vi "TSM Get PSRR Settings.vi"(0 "TSM context":T1, 11 "error in (no error)":errorcluster) -> (3 "max V":dbl format="%#_13g", 4 "TSM context Out":T1, 6 "Sampling Rate (Hz)":dbl format="%#_13g", 8 "Samples per channel":i32=1000, 14 "min V":dbl format="%#_13g", 15 "error out":errorcluster)   [LabVIEW 2020]
doc: "Gets the PSRR settings from the specification file using TSM context"
uses:
  <vilib>/NI_TestStand_SemiconductorModule/NI_TestStand_Semiconductor_Module.lvlibp/PinMap/General/SemiconductorModuleContext.ctl
  <vilib>/NI_TestStand_SemiconductorModule/NI_TestStand_Semiconductor_Module.lvlibp/PinMap/Specs/NamespacedSymbolsToValues.vi
  <vilib>/NI_TestStand_SemiconductorModule/NI_TestStand_Semiconductor_Module.lvlibp
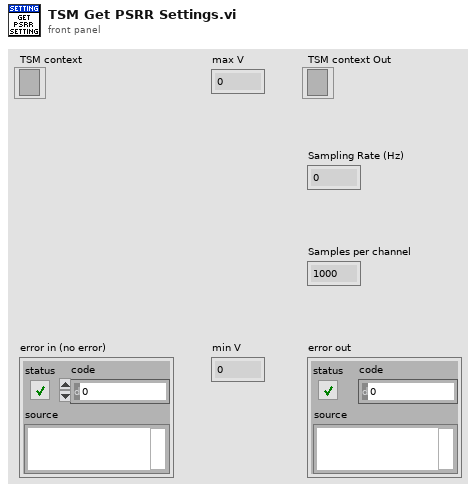
[diagram p1: front panel]
types:
  T1 = typedef "NI_TestStand_Semiconductor_Module.lvlibp/SemiconductorModuleContext.ctl" = refnum<k7>
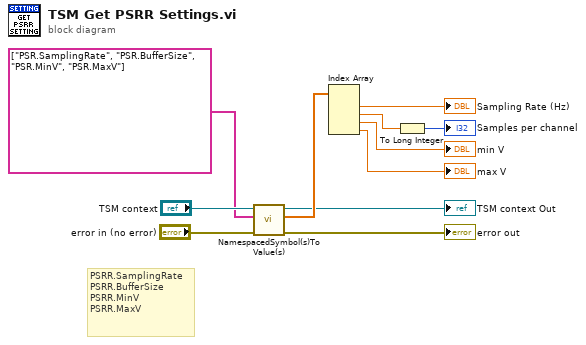
[diagram p0: block diagram]
diagram:
  # "PSRR.SamplingRate\nPSRR.BufferSize\nPSRR.MinV\nPSRR.MaxV"
  n1 = call-poly <vilib>:"NamespacedSymbol(s)ToValue(s).vi"("error in (no error)"="error in (no error)", "Symbols"=tag[] ["PSR.SamplingRate", "PSR.BufferSize", "PSR.MinV", "PSR.MaxV"], "Semiconductor Module Context"="TSM context") -> ("error out"=→"error out":errorcluster, "Values"=w8:dbl[], "Semiconductor Module Context Out"=→"TSM context Out":T1)  [unwired: 6 in]
  n2 = Index Array(array=w8) -> (element #1=→"Sampling Rate (Hz)":dbl, element #2=w2:dbl, element #3=→"min V":dbl, element #4=→"max V":dbl)  [unwired: 4 in]
  n3 = To Long Integer(number=w2) -> (32bit integer=→"Samples per channel":i32)
